vi "Controller Generate Addresses Filter Coefficients2.vi"(8 "error in (no error)":errorcluster, 9 "reset?":bool, 10 "Base address":u16, 11 "Coefficients in":fxp<+/-,22,4>[][](array[numeric])) -> (0 "error out":errorcluster, 1 "Coefficients out":fxp<+/-,22,4>[](array[numeric]), 2 "Address":u16, 3 "All coefficients loaded?":bool)   [LabVIEW 2011, in "Controller VIs.lvlib"]
uses:
  Controller VIs.lvlib
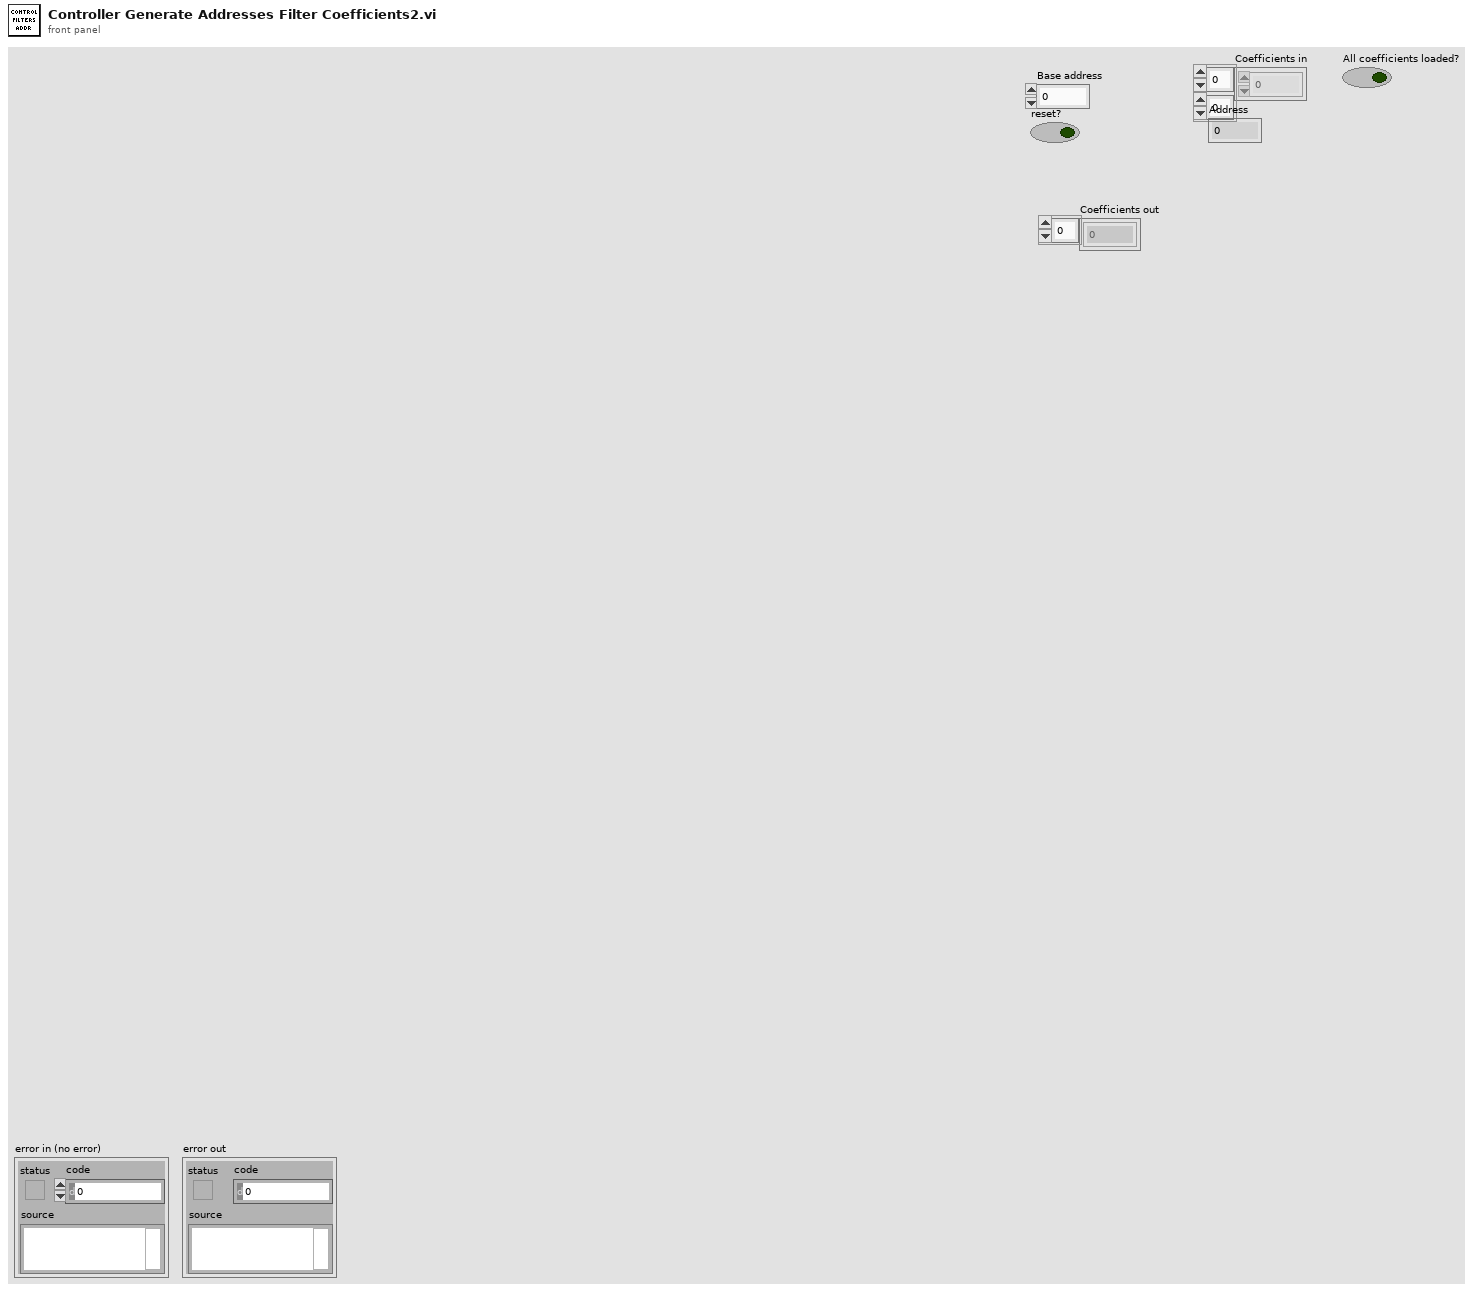
[diagram p1: front panel]
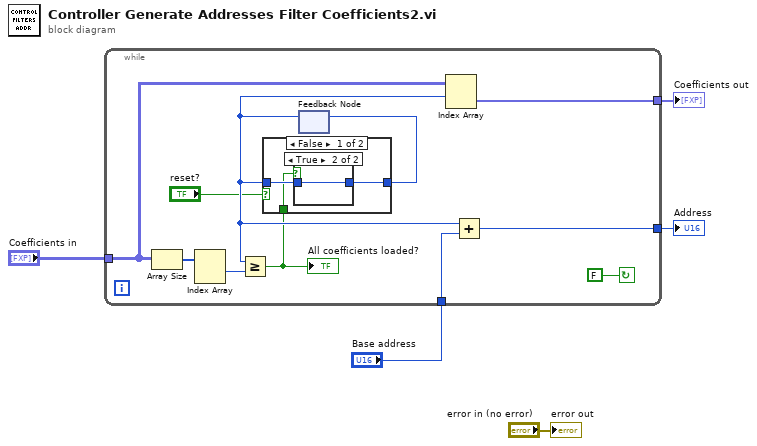
[diagram p0: block diagram]
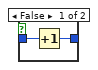
[diagram p2: hidden frame]
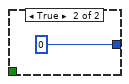
[diagram p3: hidden frame]
diagram:
  n1 = while {
    tunnel: "Coefficients in" -> [w12]
    tunnel: [w14] -> w3
    tunnel: [w13] -> w1
    tunnel: "Base address" -> [w10]
    stop <- FALSE continue-if-true
    n2 = Array Size(array=w12) -> (size(s)=w9:i32[])
    n3 = Index Array(array=w9) -> (element #1=w8:i32)  [unwired: 2 in, 1 out]
    n4 = feedback #1() -> (w11:u16)  [unwired: 1 in]
    n5 = Greater Or Equal?(x=w11, y=w8) -> (x >= y?=w6:bool)
    "All coefficients loaded?" <- w6
    n6 = case shown="False" "reset?" {
      tunnel: w11 -> [w19 _]
      tunnel: [w18 u16 0] -> w16
      tunnel: w6 -> [w17 _]
      frame False {
        n7 = case shown="True" w17 {
          tunnel: w19 -> [w21 w22]
          tunnel: [w20 w22] -> w18
          frame False {
            n8 = Increment(x=w21) -> (x+1=w20:u16)
          }
          frame True {
          }
        }
      }
      frame True {
      }
    }
    n9 = feedback-in #1(w16) -> ()
    n10 = Index Array(array=w12, index (row)=w11) -> (element=w13:fxp<+/-,22,4>[])  [unwired: 1 in]
    n11 = Add(x=w11, y=w10) -> (x+y=w14:u16)
  }
  "Address" <- w3
  "Coefficients out" <- w1
  "error out" <- "error in (no error)"
